vi "HEWH Set DRM Mode.vi"(0 "MW100":refnum<visa-resource-name>="MW100", 5 "Mode":T1 items=["CRITICAL", "HIGH", "MEDIUM", "Normal"], 11 "error in (no error)":errorcluster) -> (15 "error out":errorcluster)   [LabVIEW 2014]
uses:
  Type Definitions/Use Modes.ctl
  Type Definitions/ChannelSettings.ctl
panel:
  # "NORMAL  UNC     UNC\nMEDIUM   EHEAT UNC\nHIGH        EHEAT 110\nCRITICAL EHEAT 100"
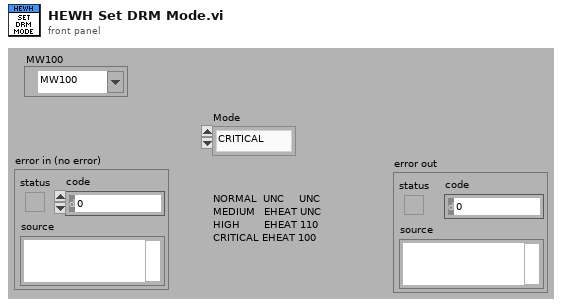
[diagram p1: front panel]
types:
  T1 = typedef "Use Modes.ctl" = u16
  T2 = typedef "ChannelSettings.ctl" = u32
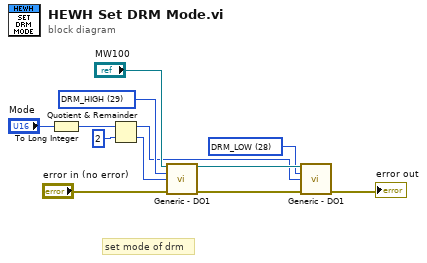
[diagram p0: block diagram]
diagram:
  w8 = T2 28 items=["4-20_OUT", "Pres_HI1", "Pres_HI2", "Pres_LOW", "Pres_PIN", "HEATER_TOP", "HEATER_BOT", "T_Shell", "FLOWMETER", "WATT_SENSE", "WH_TICK", "Tc_1", "Tc_2", "Tc_3", "Tc_4", "Tc_5", "Tc_6", "Tc_down", "T_Shell_2", "T_Shell_3", "T_Shell_4", "RTD_IN", "RTD_OUT", "RTD_AMB", "INTF_TEMPFLO", "INTF_READY", "INTF_START", "INTF_STOP", "DRM_LOW", "DRM_HIGH", "PWR_MAIN", "VLV_DUMP", "VLV_OUT", "VLV_IN", "WATT_HOURS", "FLOW(SAMPLE)", "GALLONS", "FLOW(GPM)"] ("Channel_Enum")
  w9 = T2 29 items=["4-20_OUT", "Pres_HI1", "Pres_HI2", "Pres_LOW", "Pres_PIN", "HEATER_TOP", "HEATER_BOT", "T_Shell", "FLOWMETER", "WATT_SENSE", "WH_TICK", "Tc_1", "Tc_2", "Tc_3", "Tc_4", "Tc_5", "Tc_6", "Tc_down", "T_Shell_2", "T_Shell_3", "T_Shell_4", "RTD_IN", "RTD_OUT", "RTD_AMB", "INTF_TEMPFLO", "INTF_READY", "INTF_START", "INTF_STOP", "DRM_LOW", "DRM_HIGH", "PWR_MAIN", "VLV_DUMP", "VLV_OUT", "VLV_IN", "WATT_HOURS", "FLOW(SAMPLE)", "GALLONS", "FLOW(GPM)"] ("Channel_Enum")
  # "set mode of drm"
  n1 = To Long Integer(number="Mode") -> (32bit integer=w6:i32)
  n2 = Quotient & Remainder(x=w6, y=2) -> (x-y*floor(x/y)=w4:i32, floor(x/y)=w3:i32)
  n3 = call "Generic - DO1.vi"("VISA session"="MW100", "Channel_Enum"=w9, "Relay Status (0:CLOSED)"=w3, "Error In"="error in (no error)") -> ("dup VISA session"=w12:refnum<visa-resource-name>, "error out"=w11:errorcluster)  [unwired: 10 in]
  n4 = call "Generic - DO1.vi"("VISA session"=w12, "Channel_Enum"=w8, "Relay Status (0:CLOSED)"=w4, "Error In"=w11) -> ("error out"=→"error out":errorcluster)  [unwired: 10 in, 1 out]
